vi "H036 Harsh Pandit SCADA Lab 1b Sem 6.vi"() -> ()   [LabVIEW 2022 SP3]
panel:
  out "root 2":dbl
  out "root 1":dbl
  in  "c":dbl
  in  "b":dbl
  in  "a":dbl
  # "Experiment 1b : To find roots of a quadratic equation"
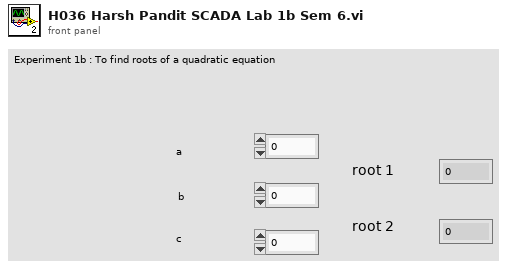
[diagram p1: front panel]
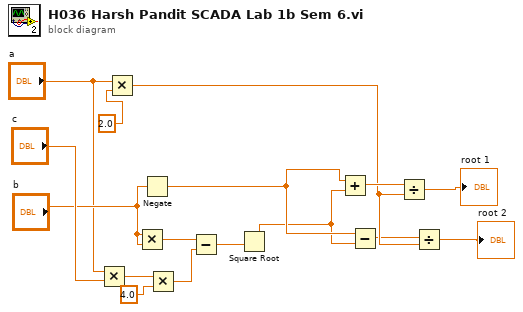
[diagram p0: block diagram]
diagram:
  n1 = Multiply(x="a", y="c") -> (x*y=w14:dbl)
  n2 = Multiply(x="a", y=2.0 ("x*y")) -> (x*y=w6:dbl)
  n3 = Multiply(x="b", y="b") -> (x*y=w16:dbl)
  n4 = Negate(x="b") -> (-x=w3:dbl)
  n5 = Multiply(x=w14, y=4.0 ("x*y")) -> (x*y=w12:dbl)
  n6 = Subtract(x=w16, y=w12) -> (x-y=w11:dbl)
  n7 = Square Root(x=w11) -> (sqrt(x)=w2:dbl)
  n8 = Add(x=w3, y=w2) -> (x+y=w7:dbl)
  n9 = Subtract(x=w3, y=w2) -> (x-y=w1:dbl)
  n10 = Divide(x=w7, y=w6) -> (x/y=→"root 1":dbl)
  n11 = Divide(x=w1, y=w6) -> (x/y=→"root 2":dbl)
